vi "DDS Startup.vi"(8 "error in (no error)":errorcluster, 11 "DDS.lvclass (in)":refnum<class "DDS.lvclass">) -> (0 "error out":errorcluster, 3 "DDS.lvclass":refnum<class "DDS.lvclass">)   [LabVIEW 2014, in "DDS.lvclass"]
uses:
  DDS.lvclass
  DDS.lvclass/DDS.ctl
  Globals.vi
  DDS Library/DDS.lvlib
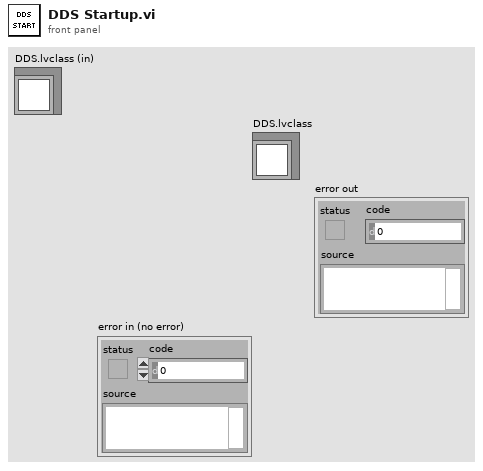
[diagram p1: front panel]
types:
  T1 = typedef "DDS.lvlib/DDS Box Array.ctl" = T2[]
  T2 = typedef "DDS.lvlib/DDS Box Cluster.ctl" = cluster{"DDS box device reference":T3, "Array of DDS Channels (4)":T5, "Enable":bool, "Description":string}
  T3 = typedef "DDS.lvlib/DDS Box Device Reference.ctl" = cluster{"NI USB-8451 device reference":T4, "DIO port":u8, "Serial Clock Rate [kHz]":u16}
  T4 = typedef "ni845xControl.ctl" = refnum<k21>
  T5 = typedef "DDS.lvlib/DDS Channel Array.ctl" = T6[]
  T6 = typedef "DDS.lvlib/DDS Channel.ctl" = cluster{"Power":bool, "Channel Parameters":T7, "RAM Enable":bool, "RAM Dest Type":T8, "RAM Default":cluster{"Frequency [MHz]":dbl, "Amplitude [dBm]":dbl, "Phase Offset [rad]":dbl}, "Array of DDS Profiles (8)":T9, "Description":string}
  T7 = typedef "DDS.lvlib/DDS Channel Parameters.ctl" = cluster{"Ref Clock Rate [MHz]":dbl, "Full Scale Output\nPower [dBm]":dbl}
  T8 = typedef "DDS.lvlib/DDS RAM Destination.ctl" = enum16{"Frequency", "Phase", "Amplitude", "Polar"}
  T9 = typedef "DDS.lvlib/DDS Profile Array.ctl" = T10[]
  T10 = typedef "DDS.lvlib/DDS Profile.ctl" = cluster{"Single Tone":cluster{"Frequency [MHz]":dbl, "Amplitude [dBm]":dbl, "Phase Offset [rad]":dbl}, "RAM Mode ":T11, "Zero-crossing":bool, "No Dwell High":bool, "Function/Static":bool, "RAM Function Settings":string[], "RAM Static Array":dbl[][], "Description":string, "Time Step (us)":T12}
  T11 = typedef "DDS.lvlib/DDS RAM mode.ctl" = enum16{"Direct Switch", "Ramp Up", "Bidirectional Ramp", "Continuous Bidirectional Ramp", "Continuous Recirculate", "Direct Switch 2", "Direct Switch 3", "Direct Switch 4"}
  T12 = typedef "DDS.lvlib/DDS RAM Timestep.ctl" = dbl
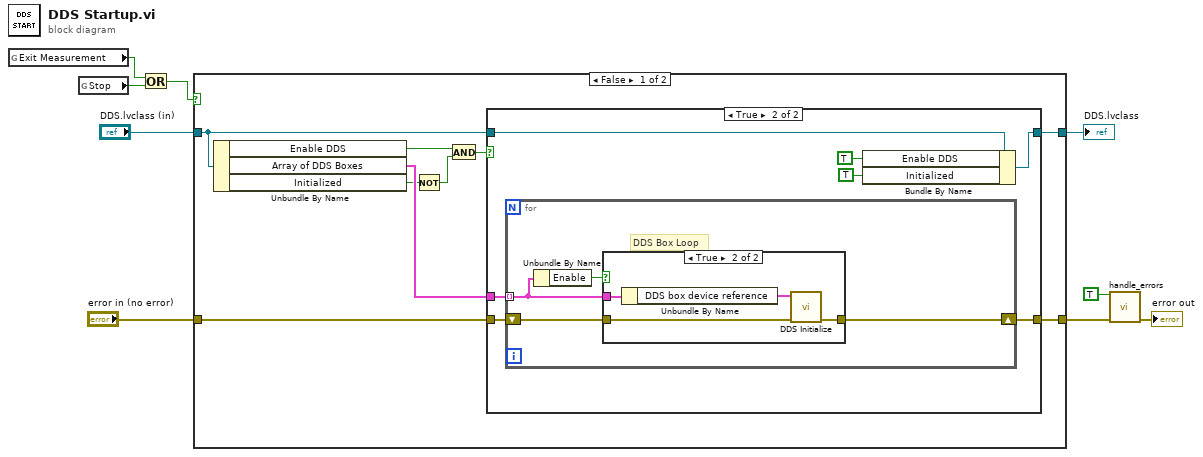
[diagram p0: block diagram]
diagram:
  n1 = global read "Globals.vi" "Exit Measurement"() -> (w7:bool)
  n2 = global read "Globals.vi" "Stop"() -> (w6:bool)
  n3 = Or(x=w7, y=w6) -> (x .or. y?=w5:bool)
  n4 = case shown="False" w5 {
    tunnel: "error in (no error)" -> [w18 w38]
    tunnel: [w16 w38] -> w2
    tunnel: "DDS.lvclass (in)" -> [w15 w37]
    tunnel: [w14 w37] -> w4
    frame False {
      n5 = Unbundle By Name(w15) -> ("Enable DDS"=w13:bool, "Array of DDS Boxes"=w17:T1, "Initialized"=w11:bool)
      n6 = Not(x=w11) -> (.not. x?=w12:bool)
      n7 = And(x=w13, y=w12) -> (x .and. y?=w10:bool)
      n8 = case shown="True" w10 {
        tunnel: [w20 w22] -> w16
        tunnel: w18 -> [w20 w27]
        tunnel: w17 -> [_ w26]
        tunnel: w15 -> [w19 w25]
        tunnel: [w19 w24] -> w14
        frame False {
        }
        frame True {
          n9 = for {
            shift-right: [w28] -> w22
            shift-left: w27 -> [w29]
            tunnel: w26 -> [w30] mode=indexing
            # "DDS Box Loop"
            n10 = Unbundle By Name(w30) -> ("Enable"=w31:bool)
            n11 = case shown="True" w31 {
              tunnel: w30 -> [_ w36]
              tunnel: w29 -> [w32 w33]
              tunnel: [w32 w34] -> w28
              frame False {
              }
              frame True {
                n12 = Unbundle By Name(w36) -> ("DDS box device reference"=w35:T3)
                n13 = call "DDS Initialize.vi"("error in (no error)"=w33, "DDS ref in"=w35) -> ("error out"=w34:errorcluster)  [unwired: 8 in, 1 out]
              }
            }
          }
          n14 = Bundle By Name(cluster=w25, "Enable DDS"=TRUE ("DDS Settings.Enable DDS"), "Initialized"=TRUE) -> (w24:refnum<class "DDS.lvclass">)
        }
      }
    }
    frame True {
    }
  }
  "DDS.lvclass" <- w4
  n15 = call "handle_errors.vi"("Exit Operation"=TRUE ("Exit Measurement"), "error in (no error)"=w2) -> ("error out"=→"error out":errorcluster)  [unwired: 13 in]
